vi "Lighting Test Software 3.vi"() -> ()   [LabVIEW 2016]
panel:
  in  "Tab Control":enum32{"Map", "Settings"}(tab)
  in  "Slide":dbl(slide) scale=0.0..1.0
  in  "Array 3":cluster{"Color Box":u32, "Slide":dbl}[][](array[cluster])=[[{"Color Box"=4934475, "Slide"=3.0}, {"Color Box"=6579300, "Slide"=4.0}, {"Color Box"=4934475, "Slide"=3.0}, {"Color Box"=4934475, "Slide"=3.0}, {"Color Box"=0, "Slide"=0.0}, {"Color Box"=0, "Slide"=0.0}], [{"Color Box"=4934475, "Slide"=3.0}, {"Color Box"=11513775, "Slide"=7.0}, {"Color Box"=8224125, "Slide"=5.0}, {"Color Box"=8224125, "Slide"=5.0}, {"Color Box"=0, "Slide"=0.0}, {"Color Box"=0, "Slide"=0.0}], [{"Color Box"=3289650, "Slide"=2.0}, {"Color Box"=3289650, "Slide"=2.0}, {"Color Box"=4934475, "Slide"=3.0}, {"Color Box"=4934475, "Slide"=3.0}, {"Color Box"=0, "Slide"=0.0}, {"Color Box"=0, "Slide"=0.0}], [{"Color Box"=8224125, "Slide"=5.0}, {"Color Box"=9868950, "Slide"=6.0}, {"Color Box"=13158600, "Slide"=8.0}, {"Color Box"=4934475, "Slide"=3.0}, {"Color Box"=0, "Slide"=0.0}, {"Color Box"=0, "Slide"=0.0}], [{"Color Box"=0, "Slide"=0.0}, {"Color Box"=0, "Slide"=0.0}, {"Color Box"=0, "Slide"=0.0}, {"Color Box"=0, "Slide"=0.0}, {"Color Box"=0, "Slide"=0.0}, {"Color Box"=0, "Slide"=0.0}], [{"Color Box"=0, "Slide"=0.0}, {"Color Box"=0, "Slide"=0.0}, {"Color Box"=0, "Slide"=0.0}, {"Color Box"=0, "Slide"=0.0}, {"Color Box"=0, "Slide"=0.0}, {"Color Box"=0, "Slide"=1.0869565217391304}]] {"Slide" min=0.0 max=10.0 scale=-1.0..11.0 scale format="%_1g"}
  in  "Save Config":bool
  in  "Load Config":bool
  in  "Index":cluster{"Numeric":i32}[][](array[cluster])=[[{"Numeric"=0}, {"Numeric"=1}, {"Numeric"=2}, {"Numeric"=3}, {"Numeric"=4}, {"Numeric"=5}], [{"Numeric"=6}, {"Numeric"=7}, {"Numeric"=8}, {"Numeric"=9}, {"Numeric"=10}, {"Numeric"=11}], [{"Numeric"=12}, {"Numeric"=-1}, {"Numeric"=-1}, {"Numeric"=13}, {"Numeric"=-1}, {"Numeric"=-1}], [{"Numeric"=14}, {"Numeric"=-2}, {"Numeric"=15}, {"Numeric"=16}, {"Numeric"=17}, {"Numeric"=18}], [{"Numeric"=19}, {"Numeric"=20}, {"Numeric"=21}, {"Numeric"=22}, {"Numeric"=-3}, {"Numeric"=-3}], [{"Numeric"=23}, {"Numeric"=-1}, {"Numeric"=-1}, {"Numeric"=24}, {"Numeric"=-3}, {"Numeric"=-3}]]
  in  "physical channels":refnum<k21>="Dev0/Ao0:15"
  in  "physical channels 2":refnum<k21>="Dev1/Ao0:15"
  out "error out":errorcluster
  out "specific error cleared?":bool
  in  "OK":bool
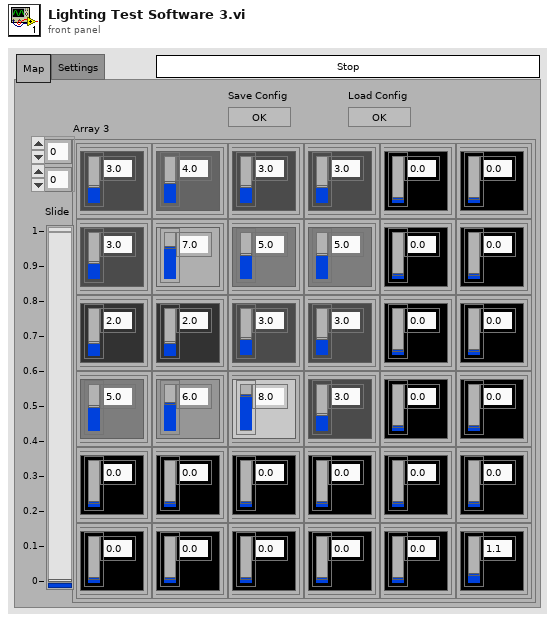
[diagram p1: front panel]
types:
  T1 = enum32{"invalid app kind", "Development System", "Run Time System", "Student Edition", "Embedded LabVIEW", "Evaluation", "Custom"}
  T2 = enum32{"Invalid", "Standard", "Closed", "Hidden", "Minimized", "Maximized"}
  T3 = cluster{"Core":cluster{"Current VI Reference":refnum<vi>, "Close Panel on Exit?":bool}, "Your Boolean data":bool}
  T4 = cluster{"Current VI Reference":refnum<vi>, "Close Panel on Exit?":bool}
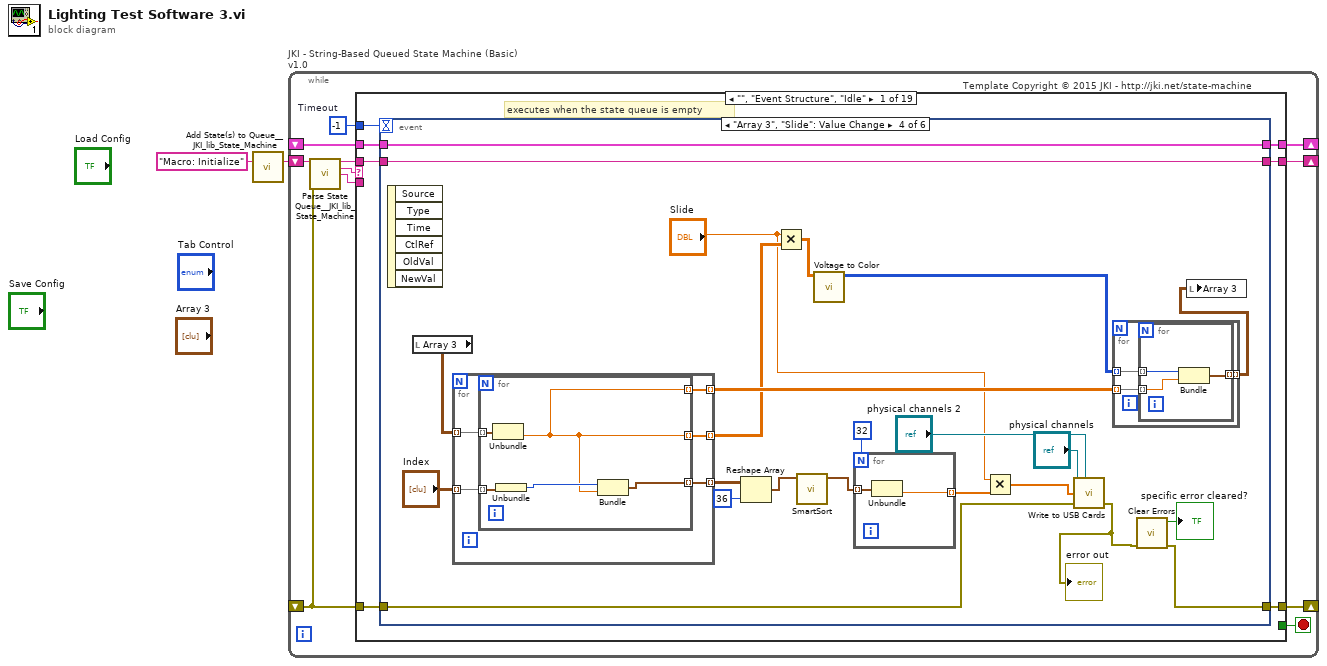
[diagram p0: block diagram]
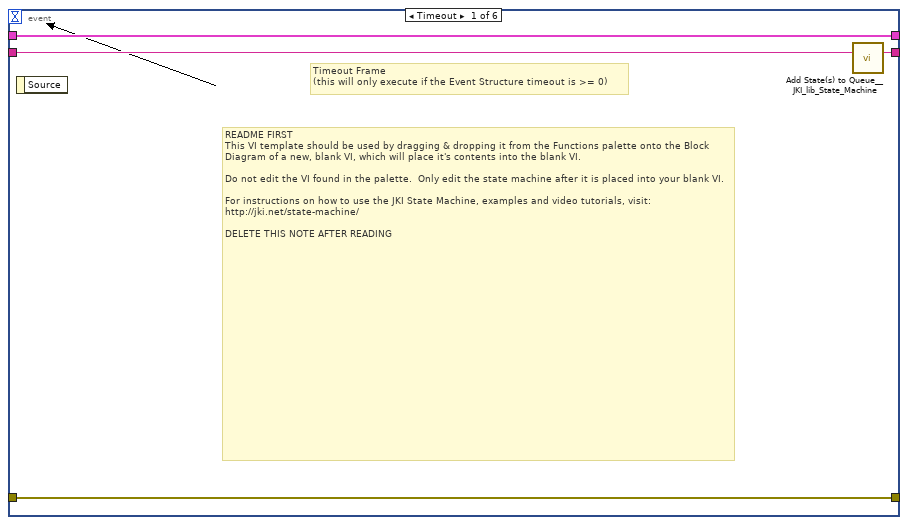
[diagram p2: hidden frame]
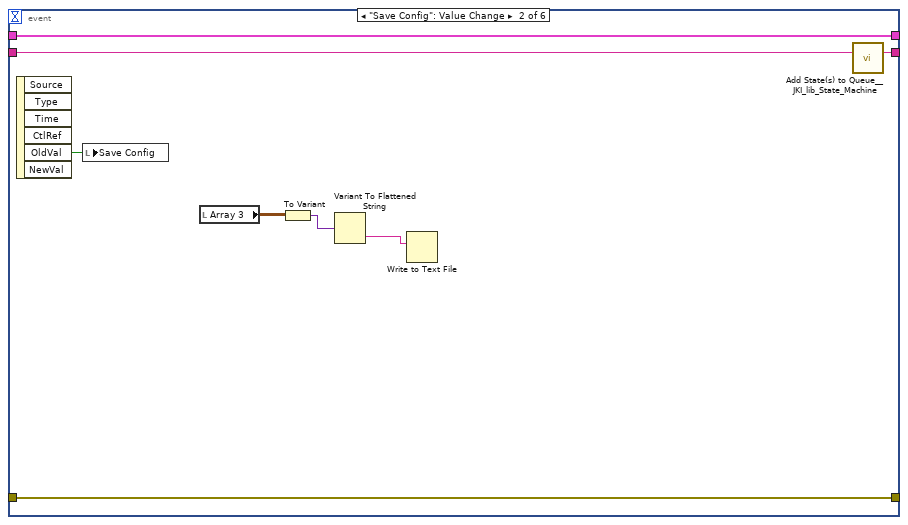
[diagram p3: hidden frame]
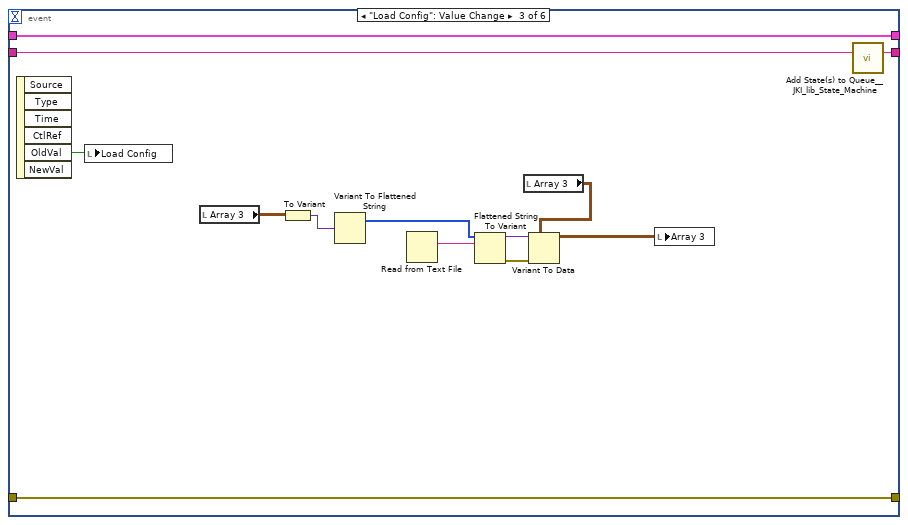
[diagram p4: hidden frame]
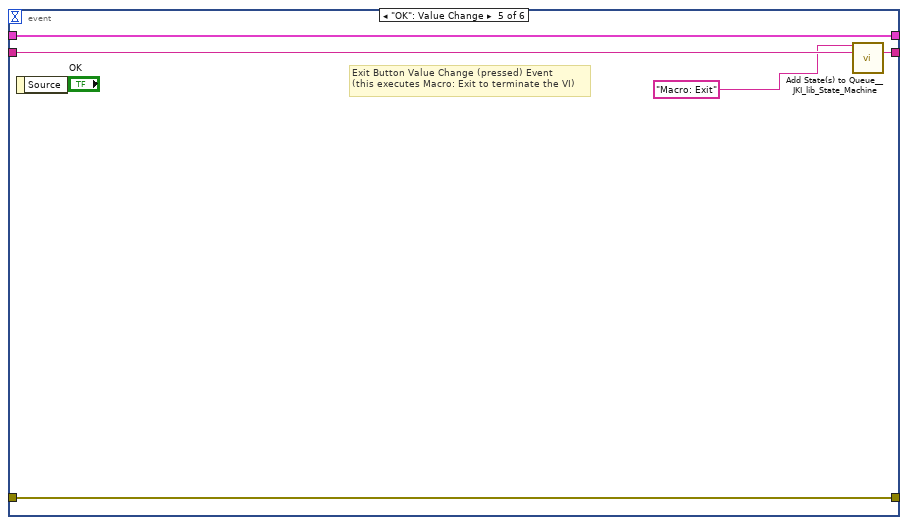
[diagram p5: hidden frame]
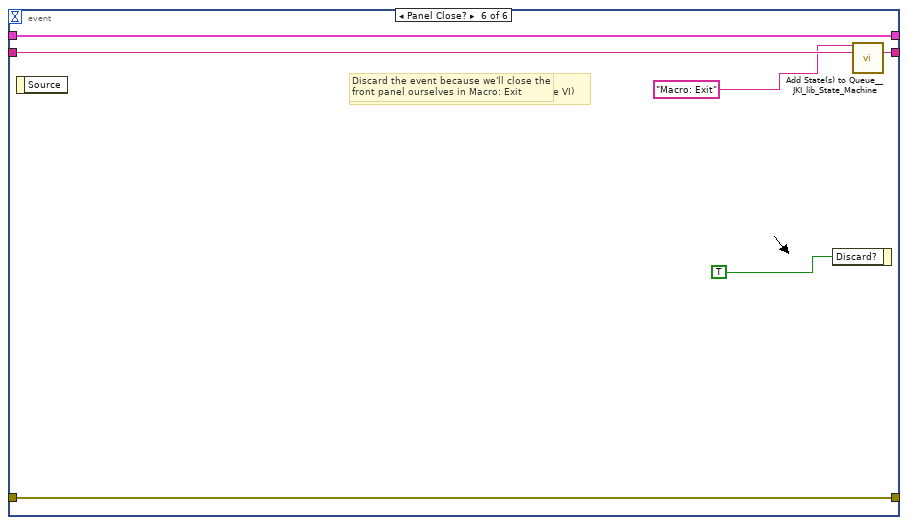
[diagram p6: hidden frame]
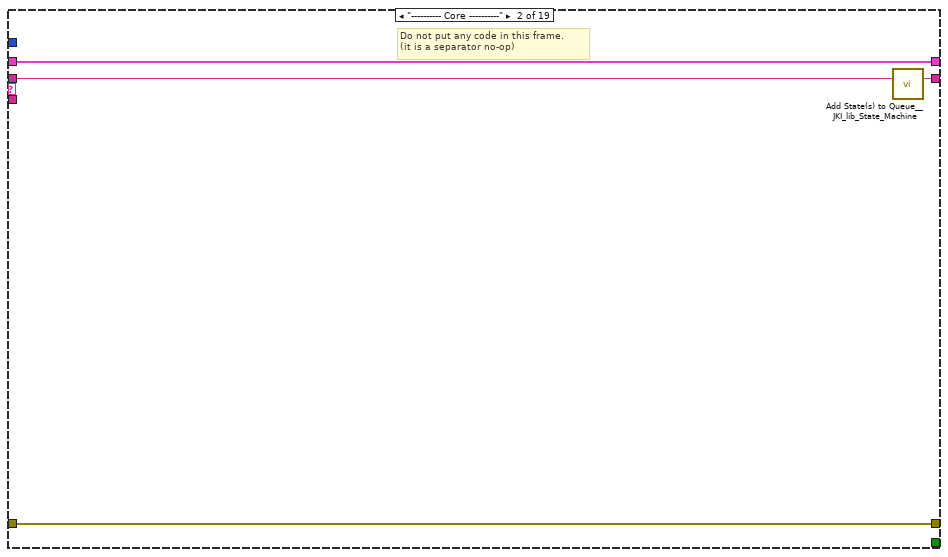
[diagram p7: hidden frame]
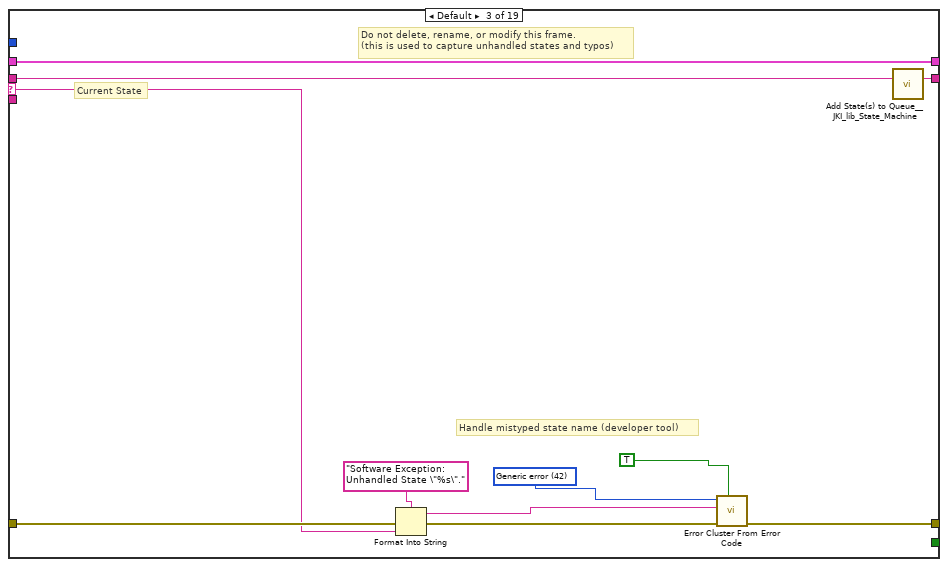
[diagram p8: hidden frame]
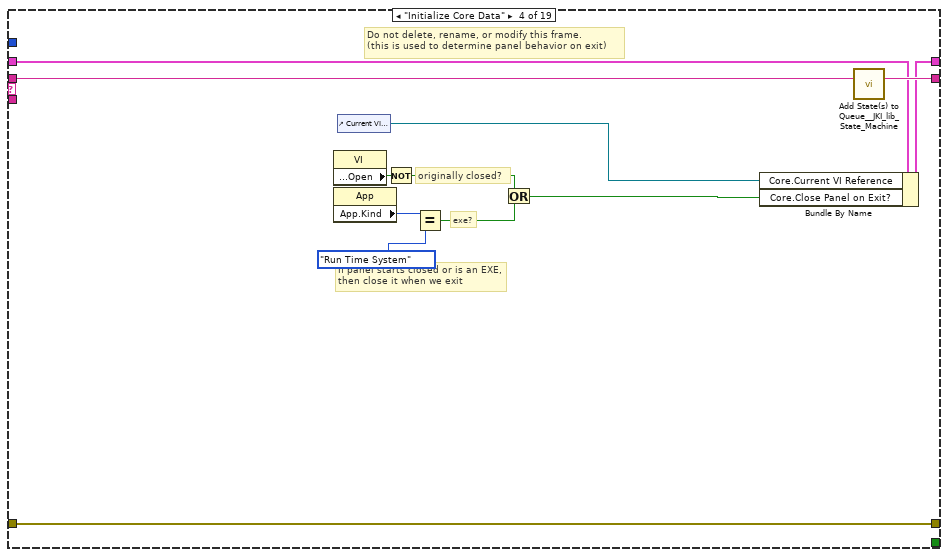
[diagram p9: hidden frame]
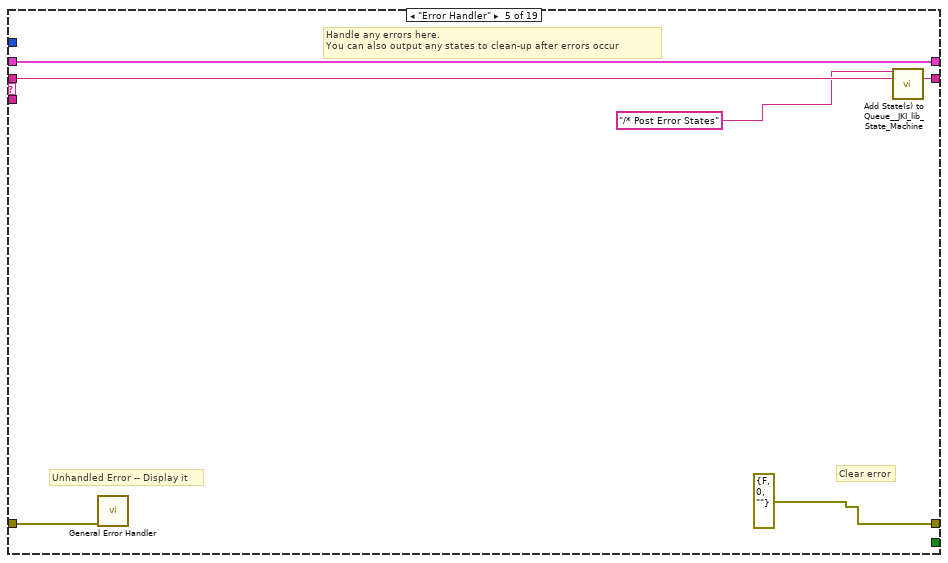
[diagram p10: hidden frame]
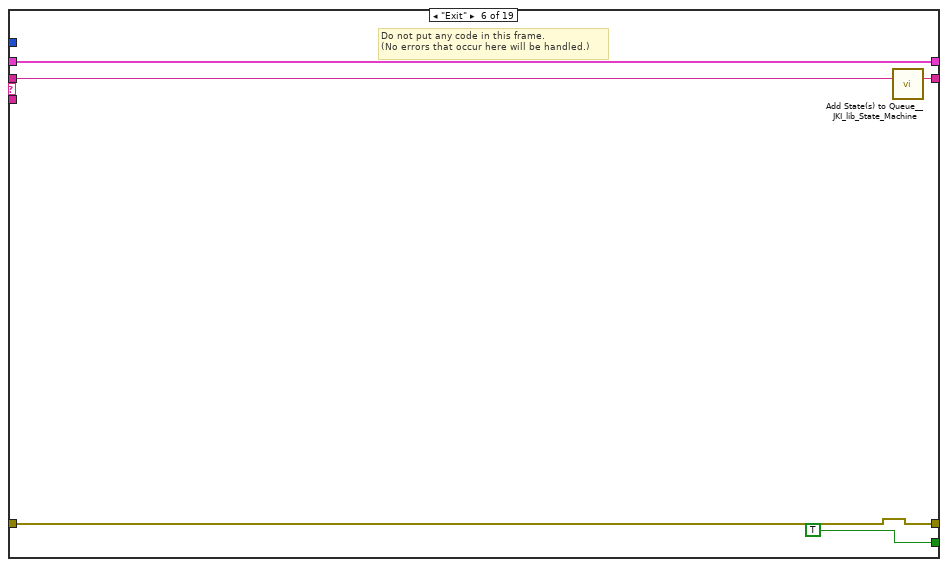
[diagram p11: hidden frame]
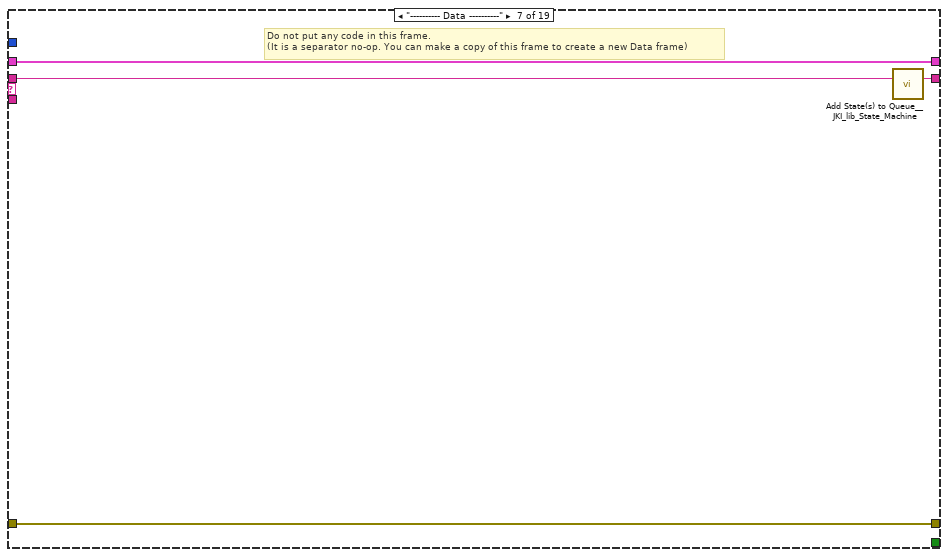
[diagram p12: hidden frame]
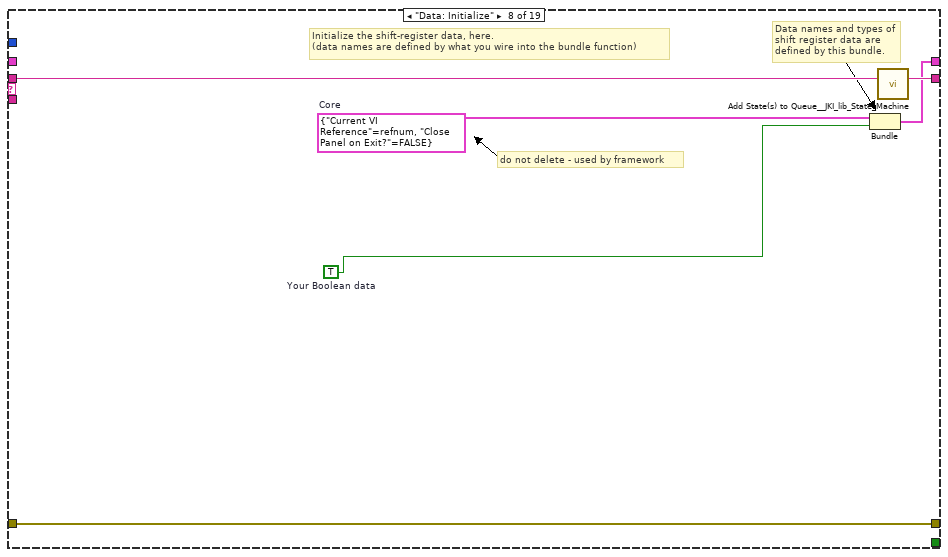
[diagram p13: hidden frame]
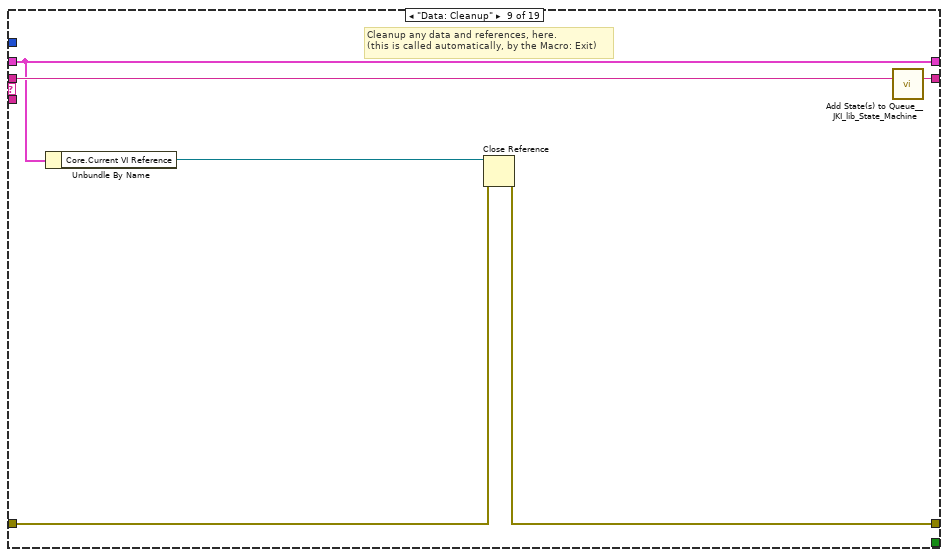
[diagram p14: hidden frame]
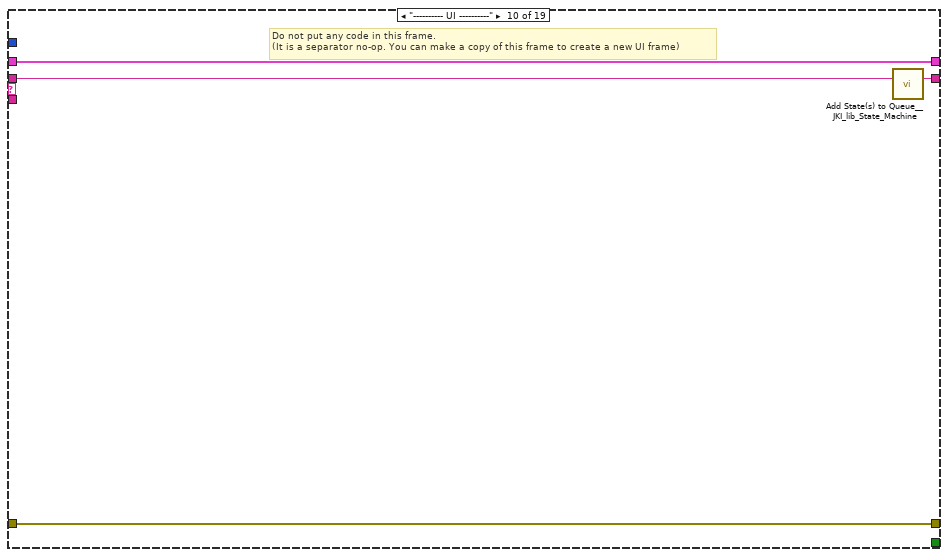
[diagram p15: hidden frame]
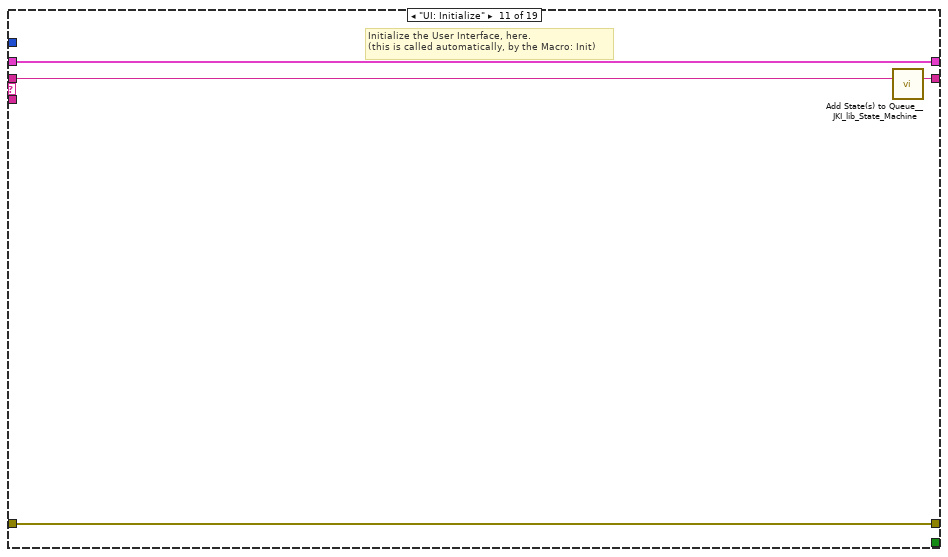
[diagram p16: hidden frame]
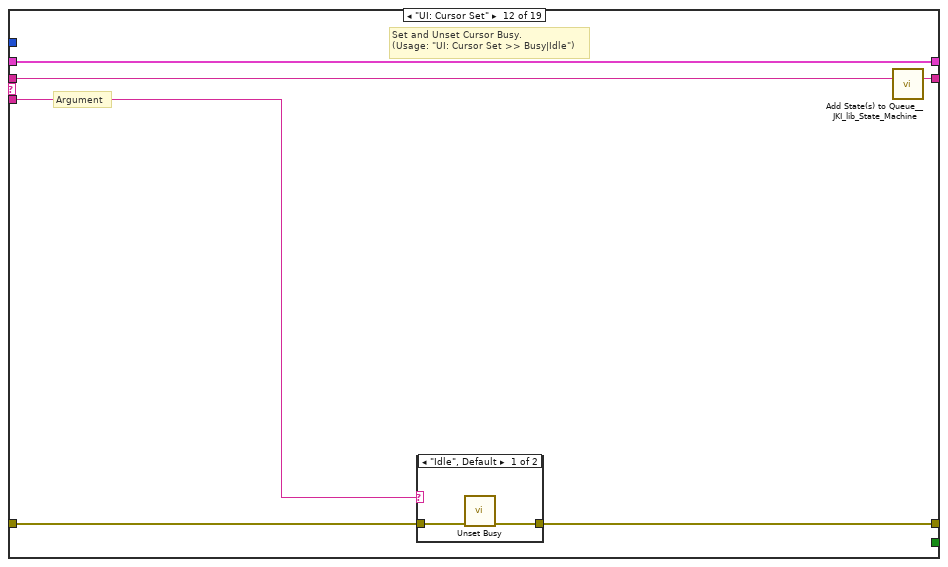
[diagram p17: hidden frame]
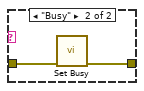
[diagram p18: hidden frame]
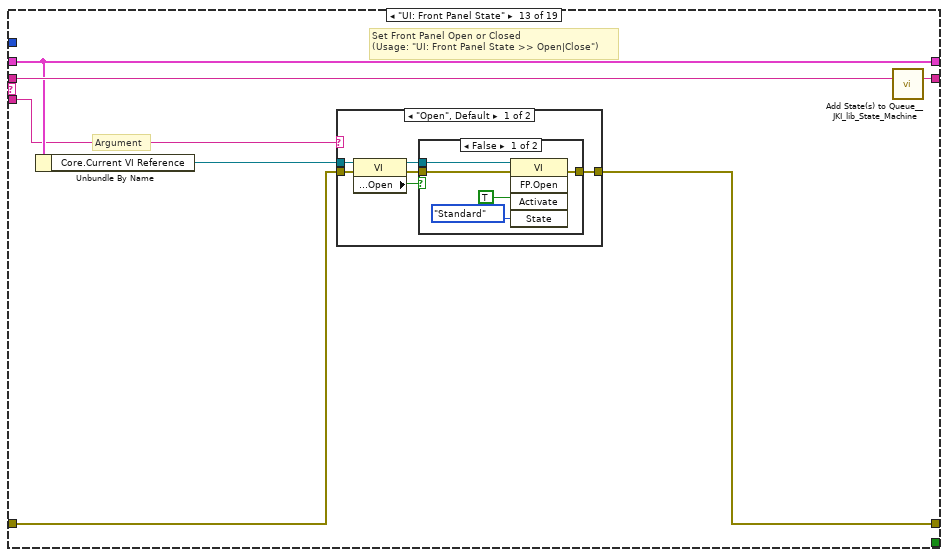
[diagram p19: hidden frame]
diagram:
  n1 = call <vilib>:"Add State(s) to Queue__JKI_lib_State_Machine.vi"("State(s) in (\"\")"="Macro: Initialize") -> ("States Out"=w2:string)  [unwired: 14 in]
  n2 = while "JKI - String-Based Queued State Machine (Basic) v1.0" {
    shift-right: [w6] -> _
    shift-left: _ -> [w5]
    shift-right: [w9] -> _
    shift-left: _ -> [w3]
    shift-right: [w8] -> _
    shift-left: w2 -> [w10]
    stop <- w7 stop-if-true
    w4 = -1  # Timeout
    # "Template Copyright © 2015 JKI - http://jki.net/state-machine"
    n3 = call <vilib>:"Parse State Queue__JKI_lib_State_Machine.vi"("State Queue"=w10, "Error In (no error)"=w3) -> ("Remaining States"=w12:string, "Current State"=w13:string, "Arguments"=w11:string)  [unwired: 11 in]
    n4 = case shown="\"\", \"Event Structure\", \"Idle\"" w13 {
      selector: w13 -> [_ _ w102 _ _ _ _ _ _ _ _ _ _ _ _ _ _ _ _]
      tunnel: w12 -> [w20 w101 w106 w124 w130 w135 w139 w145 w151 w155 w159 w165 w176 w202 w207 w217 w221 w225 w229]
      tunnel: w11 -> [_ _ _ _ _ _ _ _ _ _ _ w160 w170 _ _ _ _ _ _]
      tunnel: w5 -> [w18 w98 w104 w115 w127 w132 w136 _ w146 w152 w157 w163 w172 w199 w204 w214 w218 w222 w226]
      tunnel: [w17 w99 w108 w121 errorcluster {"status"=FALSE, "code"=0, "source"=""} ("error out") w131 w137 w140 w147 w153 w156 w161 w173 w200 w205 w215 w219 w223 w227] -> w9
      tunnel: w3 -> [w16 w99 w107 w121 w126 w131 w137 w140 w148 w153 w156 w162 w174 w200 w205 w215 w219 w223 w227]
      tunnel: [w19 w100 w105 w123 w129 w134 w138 w144 w150 w154 w158 w164 w175 w201 w206 w216 w220 w224 w228] -> w8
      tunnel: [_ _ _ _ _ TRUE _ _ _ _ _ _ _ _ _ _ _ _ _] -> w7
      tunnel: [w15 w98 w104 w122 w127 w132 w136 w143 w146 w152 w157 w163 w172 w199 w204 w214 w218 w222 w226] -> w6
      tunnel: w4 -> [w14 _ _ _ _ _ _ _ _ _ _ _ _ _ _ _ _ _ _]
      frame "", "Event Structure", "Idle" {
        # "executes when the state queue is empty"
        n5 = event shown="[3] \"Array 3\", \"Slide\": Value Change" {
          selector: _ -> [_ _ _ _ _ _]
          dyn-events: _ -> [_ _ _ _ _ _]
          timeout: w14 -> [_ _ _ _ _ _]
          tunnel: w20 -> [w24 w32 w45 w67 w91 w97]
          tunnel: [w23 w31 w44 w67 w90 w96] -> w19
          tunnel: w18 -> [w21 w29 w42 w68 w88 w94]
          tunnel: [w22 w30 w43 w53 w89 w95] -> w17
          tunnel: w16 -> [w22 w30 w43 w54 w89 w95]
          tunnel: [w21 w29 w42 w68 w88 w94] -> w15
          event Timeout {
            # "README FIRST\nThis VI template should be used by dragging & dropping it from the Functions palette onto the Block Diagram of a new, blank VI, which will place it's contents into the blank VI.\n\nDo not edit the VI found in the palette.  Only edit the state machine after it is placed into your blank VI.\n\nFor instructions on how to use the JKI State Machine, examples and video tutorials, visit:\nhttp://jki.net/state-machine/\n\nDELETE THIS NOTE AFTER READING"
            # "Timeout Frame\n(this will only execute if the Event Structure timeout is >= 0)"
            n6 = event-data() -> ()  [unwired: 1 in, 1 out]
            n7 = call <vilib>:"Add State(s) to Queue__JKI_lib_State_Machine.vi"("State(s) in (\"\")"=w24) -> ("States Out"=w23:string)  [unwired: 14 in]
          }
          event "Save Config": Value Change {
            n8 = event-data() -> ("OldVal"=w25:bool)  [unwired: 1 in, 5 out]
            n9 = local write "Save Config"(w25) -> ()
            n10 = local read "Array 3"() -> (w28:cluster{"Color Box":u32, "Slide":dbl}[][])
            n11 = To Variant(anything=w28) -> (Variant=w27:variant)
            n12 = Variant To Flattened String(Variant=w27) -> (data string=w26:string)  [unwired: 1 out]
            n13 = Write to Text File(text=w26) -> ()  [unwired: 3 in, 3 out]
            n14 = call <vilib>:"Add State(s) to Queue__JKI_lib_State_Machine.vi"("State(s) in (\"\")"=w32) -> ("States Out"=w31:string)  [unwired: 14 in]
          }
          event "Load Config": Value Change {
            n15 = event-data() -> ("OldVal"=w33:bool)  [unwired: 1 in, 5 out]
            n16 = local write "Load Config"(w33) -> ()
            n17 = local read "Array 3"() -> (w41:cluster{"Color Box":u32, "Slide":dbl}[][])
            n18 = To Variant(anything=w41) -> (Variant=w36:variant)
            n19 = Variant To Flattened String(Variant=w36) -> (1:w39:i16[])  [unwired: 1 out]
            n20 = Read from Text File() -> (text=w40:string)  [unwired: 4 in, 3 out]
            n21 = Flattened String To Variant(6:w40, 7:w39) -> (0:w38:errorcluster, 3:w37:variant)  [unwired: 1 in]
            n22 = local read "Array 3"() -> (w34:cluster{"Color Box":u32, "Slide":dbl}[][])
            n23 = Variant To Data(error in=w38, type=w34, Variant=w37) -> (data=w35:cluster{"Color Box":u32, "Slide":dbl}[][])  [unwired: 1 out]
            n24 = local write "Array 3"(w35) -> ()
            n25 = call <vilib>:"Add State(s) to Queue__JKI_lib_State_Machine.vi"("State(s) in (\"\")"=w45) -> ("States Out"=w44:string)  [unwired: 14 in]
          }
          event "Array 3", "Slide": Value Change {
            n26 = event-data() -> ()  [unwired: 1 in, 6 out]
            n27 = local read "Array 3"() -> (w66:cluster{"Color Box":u32, "Slide":dbl}[][])
            n28 = for {
              tunnel: w66 -> [w81] mode=indexing
              tunnel: [w80] -> w50 mode=indexing
              tunnel: [w79] -> w63 mode=indexing
              tunnel: "Index" -> [w78] mode=indexing
              tunnel: [w77] -> w61 mode=indexing
              n29 = for {
                tunnel: w81 -> [w86] mode=indexing
                tunnel: [w83] -> w80 mode=indexing
                tunnel: [w83] -> w79 mode=indexing
                tunnel: w78 -> [w85] mode=indexing
                tunnel: [w82] -> w77 mode=indexing
                n30 = Unbundle(w86) -> ("Slide"=w83:dbl)  [unwired: 1 out]
                n31 = Unbundle(w85) -> ("Numeric"=w84:i32)
                n32 = Bundle("Numeric"=w84, "Slide"=w83) -> (w82:cluster{"Numeric":i32, "Slide":dbl})  [unwired: 1 in]
              }
            }
            n33 = Reshape Array(w61, 36 ("dimension size")) -> (w59:cluster{"Numeric":i32, "Slide":dbl}[])
            n34 = Multiply(x="Slide", y=w50) -> (x*y=w49:dbl[][])
            n35 = call "SmartSort.vi"("Array in"=w59) -> ("Array out"=w58:cluster{"Numeric":i32, "Slide":dbl}[])  [unwired: 10 in]
            n36 = call "Voltage to Color.vi"("Array in"=w49) -> ("Array out"=w64:u32[][])  [unwired: 10 in]
            n37 = for {
              N: 32 -> [_]
              tunnel: w58 -> [w70] mode=indexing
              tunnel: [w69] -> w48 mode=indexing
              n38 = Unbundle(w70) -> ("Slide"=w69:dbl)  [unwired: 1 out]
            }
            n39 = Multiply(x="Slide", y=w48) -> (x*y=w46:dbl[])
            n40 = call "Write to USB Cards.vi"("physical channels"="physical channels", "physical channels 2"="physical channels 2", "Array"=w46, "error in"=w54) -> ("error out"=w51:errorcluster)  [unwired: 5 in]
            "error out" <- w51
            n41 = for {
              tunnel: [w73] -> w65 mode=indexing
              tunnel: w64 -> [w72] mode=indexing
              tunnel: w63 -> [w71] mode=indexing
              n42 = for {
                tunnel: [w76] -> w73 mode=indexing
                tunnel: w72 -> [w75] mode=indexing
                tunnel: w71 -> [w74] mode=indexing
                n43 = Bundle(w75, "Slide"=w74) -> (w76:cluster{u32, "Slide":dbl})  [unwired: 1 in]
              }
            }
            n44 = call <vilib>:"Clear Errors.vi"("error in (no error)"=w51) -> ("error out"=w53:errorcluster, "specific error cleared?"=→"specific error cleared?":bool)  [unwired: 5 in]
            n45 = local write "Array 3"(w65) -> ()
          }
          event "OK": Value Change {
            # "Exit Button Value Change (pressed) Event\n(this executes Macro: Exit to terminate the VI)"
            n46 = event-data() -> ()  [unwired: 1 in, 1 out]
            n47 = call <vilib>:"Add State(s) to Queue__JKI_lib_State_Machine.vi"("State(s) in Front (\"\")"="Macro: Exit", "State(s) in (\"\")"=w91) -> ("States Out"=w90:string)  [unwired: 13 in]
          }
          event Panel Close? {
            # "Discard the event because we'll close the front panel ourselves in Macro: Exit"
            # "Close Panel button (pressed) Event\n(this executes Macro: Exit to terminate the VI)"
            n48 = event-data() -> ()  [unwired: 1 in, 1 out]
            n49 = event-data("Discard?"=TRUE) -> ()  [unwired: 1 in, 1 out]
            n50 = call <vilib>:"Add State(s) to Queue__JKI_lib_State_Machine.vi"("State(s) in Front (\"\")"="Macro: Exit", "State(s) in (\"\")"=w97) -> ("States Out"=w96:string)  [unwired: 13 in]
          }
        }
      }
      frame "---------- Core ----------" {
        # "Do not put any code in this frame.\n(it is a separator no-op)"
        n51 = call <vilib>:"Add State(s) to Queue__JKI_lib_State_Machine.vi"("State(s) in (\"\")"=w101) -> ("States Out"=w100:string)  [unwired: 14 in]
      }
      frame Default {
        w111 = 42 items=["No error", "Argument error", "Memory is full", "Out of zone", "End of file", "File already open", "Generic file I/O error", "File not found", "File permission error", "Disk is full", "Duplicate path", "Too many files open", "System feature not enabled", "Resource file not found", "Cannot add resource", "Resource not found", "Image not found", "Image memory error", "Pen does not exist", "Config type invalid", "Config token not found", "Config parse error", "Config memory error", "Bad external code format", "Bad external code offset", "External code not present", "Null window", "Destroy window error", "Null menu", "Print aborted", "Bad print record", "Print driver error", "Windows error during printing", "Memory error during printing", "Print dialog error", "Generic print error", "Invalid device refnum", "Device not found", "Device parameter error", "Device unit error", "Cannot open device", "Device call aborted", "Generic error", "Cancelled by user", "Object ID too low", "Object ID too high", "Object not in heap", "Unknown heap", "Unknown object (invalid DefProc)", "Unknown object (DefProc not in table)", "Message out of range", "Invalid (null) method", "Unknown message", "Manager call not supported", "Bad address", "Network operation in progress", "Network operation timed out", "Connection is busy", "Network attribute not supported", "Network error", "Address in use", "System out of memory", "Connection aborted", "Connection refused", "Not connected", "Already connected", "Connection closed", "Initialization error (interapplication manager)", "Bad occurrence", "Wait on unbound occurrence handler", "Occurrence queue overflow", "Datalog type conflict", "Unused", "Unrecognized type (interapplication manager)", "Memory corrupt", "Failed to make temporary DLL", "Old CIN version", "Drag socket not found", "Failed to load drop-object", "Failed to register OLE object", "Failed to release OLE object", "Format specifier type mismatch", "Unknown format specifier", "Too few format specifiers", "Too many format specifiers", "Scan failed", "Newer CIN version", "Error converting to variant", "Runtime menu error", "Password tampered", "Variant attribute not found", "Incompatible variant data type", "Event data is not available", "Event Store is not present", "Occurrence is not found", "Event Queue is not created", "Event info is not available", "Refnum passed is NULL", "Error retrieving Class GUID", "Error retrieving CoClass GUID", "Error retrieving TypeLib GUID.", "Bad built application magic bytes.", "Specific driver is different from the specific driver associated with the Logical Name.", "There is no session opened to the class driver.", "Max Error", "MAX - Error with config objects", "MAX - Error loading configuration", "MAX - Group not supported"]
        # "Current State"
        # "Do not delete, rename, or modify this frame.\n(this is used to capture unhandled states and typos)"
        # "Handle mistyped state name (developer tool)"
        n52 = Format Into String(format string="Software Exception: Unhandled State \"%s\"." ("message"), error in=w107, w102) -> (resulting string=w110:string, error out=w109:errorcluster)  [unwired: 1 in]
        n53 = call <vilib>:"Error Cluster From Error Code.vi"("show call chain? (False)"=TRUE, "error in (no error)"=w109, "error message (\"\")"=w110, "error code (0)"=w111) -> ("error out"=w108:errorcluster)  [unwired: 5 in]
        n54 = call <vilib>:"Add State(s) to Queue__JKI_lib_State_Machine.vi"("State(s) in (\"\")"=w106) -> ("States Out"=w105:string)  [unwired: 14 in]
      }
      frame "Initialize Core Data" {
        # "Do not delete, rename, or modify this frame.\n(this is used to determine panel behavior on exit)"
        # "originally closed?"
        # "exe?"
        # "If panel starts closed or is an EXE, then close it when we exit"
        n55 = property class="VI"() -> ("Front Panel.Open"=w120:bool)  [unwired: 2 in, 2 out]
        n56 = property class="App"() -> ("App.Kind"=w119:T1)  [unwired: 2 in, 2 out]
        n57 = control-ref of="Current VI Reference"() -> (w113:refnum<vi>)
        n58 = Not(x=w120) -> (.not. x?=w117:bool)
        n59 = Equal?(x=w119, y=T1."Run Time System" ("Application:Kind")) -> (x = y?=w116:bool)
        n60 = Or(x=w117, y=w116) -> (x .or. y?=w114:bool)
        n61 = Bundle By Name(cluster=w115, "Core.Current VI Reference"=w113, "Core.Close Panel on Exit?"=w114) -> (w122:T3)
        n62 = call <vilib>:"Add State(s) to Queue__JKI_lib_State_Machine.vi"("State(s) in (\"\")"=w124) -> ("States Out"=w123:string)  [unwired: 14 in]
      }
      frame "Error Handler" {
        # "Unhandled Error -- Display it"
        # "Handle any errors here.\nYou can also output any states to clean-up after errors occur"
        # "Clear error"
        n63 = call <vilib>:"General Error Handler.vi"("error in (no error)"=w126) -> ()  [unwired: 10 in, 5 out]
        n64 = call <vilib>:"Add State(s) to Queue__JKI_lib_State_Machine.vi"("State(s) in Front (\"\")"="/* Post Error States", "State(s) in (\"\")"=w130) -> ("States Out"=w129:string)  [unwired: 13 in]
      }
      frame "Exit" {
        # "Do not put any code in this frame.\n(No errors that occur here will be handled.)"
        n65 = call <vilib>:"Add State(s) to Queue__JKI_lib_State_Machine.vi"("State(s) in (\"\")"=w135) -> ("States Out"=w134:string)  [unwired: 14 in]
      }
      frame "---------- Data ----------" {
        # "Do not put any code in this frame.\n(It is a separator no-op. You can make a copy of this frame to create a new Data frame)"
        n66 = call <vilib>:"Add State(s) to Queue__JKI_lib_State_Machine.vi"("State(s) in (\"\")"=w139) -> ("States Out"=w138:string)  [unwired: 14 in]
      }
      frame "Data: Initialize" {
        w141 = T4 {"Current VI Reference"=refnum, "Close Panel on Exit?"=FALSE}  # Core
        w142 = TRUE  # Your Boolean data
        # "do not delete - used by framework"
        # "Data names and types of shift register data are defined by this bundle."
        # "Initialize the shift-register data, here.\n(data names are defined by what you wire into the bundle function)"
        n67 = Bundle("Core"=w141, "Your Boolean data"=w142) -> (w143:T3)  [unwired: 1 in]
        n68 = call <vilib>:"Add State(s) to Queue__JKI_lib_State_Machine.vi"("State(s) in (\"\")"=w145) -> ("States Out"=w144:string)  [unwired: 14 in]
      }
      frame "Data: Cleanup" {
        # "Cleanup any data and references, here.\n(this is called automatically, by the Macro: Exit)"
        n69 = Unbundle By Name(w146) -> ("Core.Current VI Reference"=w149:refnum<vi>)
        n70 = Close Reference(reference=w149, error in (no error)=w148) -> (error out=w147:errorcluster)
        n71 = call <vilib>:"Add State(s) to Queue__JKI_lib_State_Machine.vi"("State(s) in (\"\")"=w151) -> ("States Out"=w150:string)  [unwired: 14 in]
      }
      frame "---------- UI ----------" {
        # "Do not put any code in this frame.\n(It is a separator no-op. You can make a copy of this frame to create a new UI frame)"
        n72 = call <vilib>:"Add State(s) to Queue__JKI_lib_State_Machine.vi"("State(s) in (\"\")"=w155) -> ("States Out"=w154:string)  [unwired: 14 in]
      }
      frame "UI: Initialize" {
        # "Initialize the User Interface, here.\n(this is called automatically, by the Macro: Init)"
        n73 = call <vilib>:"Add State(s) to Queue__JKI_lib_State_Machine.vi"("State(s) in (\"\")"=w159) -> ("States Out"=w158:string)  [unwired: 14 in]
      }
      frame "UI: Cursor Set" {
        # "Argument"
        # "Set and Unset Cursor Busy.\n(Usage: \"UI: Cursor Set >> Busy|Idle\")"
        n74 = case shown="\"Idle\", Default" w160 {
          tunnel: w162 -> [w167 w169]
          tunnel: [w166 w168] -> w161
          frame "Idle", Default {
            n75 = call <vilib>:"Unset Busy.vi"("error in (no error)"=w167) -> ("error out"=w166:errorcluster)  [unwired: 10 in]
          }
          frame "Busy" {
            n76 = call <vilib>:"Set Busy.vi"("error in (no error)"=w169) -> ("error out"=w168:errorcluster)  [unwired: 9 in, 1 out]
          }
        }
        n77 = call <vilib>:"Add State(s) to Queue__JKI_lib_State_Machine.vi"("State(s) in (\"\")"=w165) -> ("States Out"=w164:string)  [unwired: 14 in]
      }
      frame "UI: Front Panel State" {
        # "Argument"
        # "Set Front Panel Open or Closed\n(Usage: \"UI: Front Panel State >> Open|Close\")"
        n78 = Unbundle By Name(w172) -> ("Core.Current VI Reference"=w171:refnum<vi>)
        n79 = case shown="\"Open\", Default" w170 {
          tunnel: w174 -> [w180 w193]
          tunnel: [w182 w194] -> w173
          tunnel: w171 -> [w181 w191]
          frame "Open", Default {
            n80 = property class="VI"(reference=w181, error in=w180) -> (reference out=w178:refnum<vi>, error out=w179:errorcluster, "Front Panel.Open"=w177:bool)
            n81 = case shown="False" w177 {
              tunnel: [w185 w188] -> w182
              tunnel: w179 -> [w184 w188]
              tunnel: w178 -> [w183 _]
              frame False {
                n82 = invoke class="VI" method="FP.Open"(reference=w183, error in=w184, "Activate"=TRUE, "State"=T2."Standard") -> (error out=w185:errorcluster)  [unwired: 1 in, 4 out]
              }
              frame True {
              }
            }
          }
          frame "Close" {
            n83 = property class="VI"(reference=w191, error in=w193) -> (reference out=w190:refnum<vi>, error out=w192:errorcluster, "Front Panel.Open"=w189:bool)
            n84 = case shown="True" w189 {
              tunnel: [w195 w198] -> w194
              tunnel: w192 -> [w195 w197]
              tunnel: w190 -> [_ w196]
              frame False {
              }
              frame True {
                n85 = invoke class="VI" method="FP.Close"(reference=w196, error in=w197) -> (error out=w198:errorcluster)  [unwired: 1 in, 2 out]
              }
            }
          }
        }
        n86 = call <vilib>:"Add State(s) to Queue__JKI_lib_State_Machine.vi"("State(s) in (\"\")"=w176) -> ("States Out"=w175:string)  [unwired: 14 in]
      }
      frame "---------- Macro ----------" {
        # "Do not put any code in this frame.\n(It is a separator no-op. You can make a copy of this frame to create a new Macro frame)"
        n87 = call <vilib>:"Add State(s) to Queue__JKI_lib_State_Machine.vi"("State(s) in (\"\")"=w202) -> ("States Out"=w201:string)  [unwired: 14 in]
      }
      frame "Macro: Initialize" {
        w203 = "Data: Initialize\nInitialize Core Data\nUI: Initialize\nUI: Front Panel State >> Open"  # Data: Initialize Initialize Core Data UI: Initialize UI: Front Panel State >> Open
        # "Initialization Macro\n(This is called once, when the VI starts)"
        n88 = call <vilib>:"Add State(s) to Queue__JKI_lib_State_Machine.vi"("State(s) in Front (\"\")"=w203, "State(s) in (\"\")"=w207) -> ("States Out"=w206:string)  [unwired: 13 in]
      }
      frame "Macro: Exit" {
        # "Exit Macro\n(This is called once, when the VI exits)"
        n89 = Unbundle By Name(w214) -> ("Core.Close Panel on Exit?"=w213:bool)
        n90 = Select(t="UI: Front Panel State >> Close", s=w213, f="") -> (s? t:f=w210:string)
        n91 = call <vilib>:"Add State(s) to Queue__JKI_lib_State_Machine.vi"("State(s) in (\"\")"=w210, "State(s) at Back (\"\")"="Data: Cleanup\nExit") -> ("States Out"=w208:string)  [unwired: 13 in]
        n92 = call <vilib>:"Add State(s) to Queue__JKI_lib_State_Machine.vi"("State(s) in Front (\"\")"=w208, "State(s) in (\"\")"=w217) -> ("States Out"=w216:string)  [unwired: 13 in]
      }
      frame "---------- New Category ----------" {
        # "Template Separator\n(You can make a copy of, or modify, this frame)"
        n93 = call <vilib>:"Add State(s) to Queue__JKI_lib_State_Machine.vi"("State(s) in (\"\")"=w221) -> ("States Out"=w220:string)  [unwired: 14 in]
      }
      frame "New Category: 1" {
        # "Your code here.\n(You can make a copy of, or modify, this frame)"
        n94 = call <vilib>:"Add State(s) to Queue__JKI_lib_State_Machine.vi"("State(s) in (\"\")"=w225) -> ("States Out"=w224:string)  [unwired: 14 in]
      }
      frame "New Category: 2" {
        # "Your code here.\n(You can make a copy of, or modify, this frame)"
        n95 = call <vilib>:"Add State(s) to Queue__JKI_lib_State_Machine.vi"("State(s) in (\"\")"=w229) -> ("States Out"=w228:string)  [unwired: 14 in]
      }
    }
  }
